vi "LCP Get Next Dosage Time.vi"(8 "error in (no error)":errorcluster caption="Fehler (Eingang, kein Fehler)", 11 "hPump":i32) -> (0 "error out":errorcluster caption="Fehler (Ausgang)", 3 "function return":i32)   [LabVIEW 2010, in "labbCAN_Pump_API.lvlib"]
doc: "LCP_Func long LCP_CALL LCP_GetNextDosageTime(dev_hdl hPump);"
uses:
  labbCAN_Pump_API.lvlib
  labbCAN_Pump_API.dll
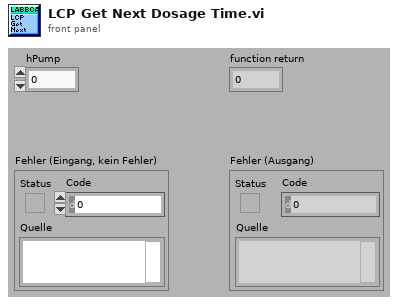
[diagram p1: front panel]
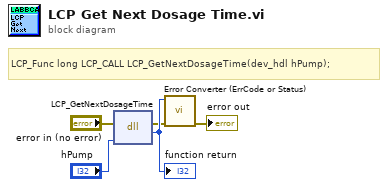
[diagram p0: block diagram]
diagram:
  # "LCP_Func long LCP_CALL LCP_GetNextDosageTime(dev_hdl hPump);"
  n1 = dll-call lib="C:/CodingXP/cetoni_projects/QmixSDK/labbCAN_Pump_API.*" fn="LCP_GetNextDosageTime"(error in="error in (no error)", "hPump"="hPump") -> (error out=w2:errorcluster, w5:i32)  [unwired: 3 in, 1 out]
  "function return" <- w5
  n2 = call "Error Converter (ErrCode or Status).vi"("error in (no error)"=w2, "error code"=w5) -> ("error out"=→"error out":errorcluster)  [unwired: 9 in]
